vi "read_probes.vi"(8 "error in (no error)":errorcluster, 11 "TempProbeSet in":refnum<class "TempProbeSet.lvclass">) -> (0 "error out":errorcluster, 2 "Array":refnum<class "TempProbe.lvclass">[](array[class]), 3 "TempProbeSet out":refnum<class "TempProbeSet.lvclass">)   [LabVIEW 2010, in "TempProbeSet.lvclass"]
uses:
  TempProbeSet.lvclass
  TempProbe.lvclass
  TempProbeSet.lvclass/TempProbeSet.ctl
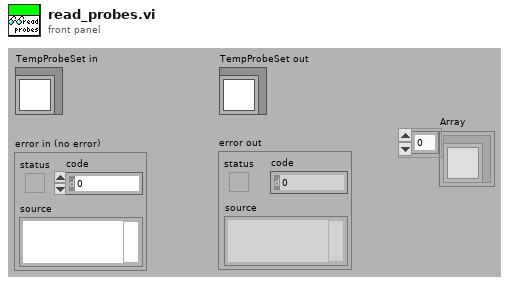
[diagram p1: front panel]
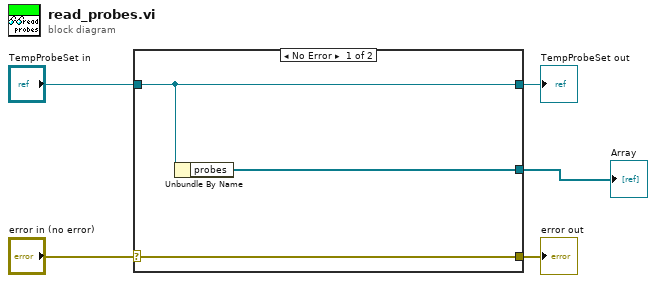
[diagram p0: block diagram]
diagram:
  n1 = case shown="No Error" "error in (no error)" {
    selector: "error in (no error)" -> [w8 w9]
    tunnel: [w8 w9] -> w4
    tunnel: [w7 w10] -> w2
    tunnel: "TempProbeSet in" -> [w7 w10]
    tunnel: [w6 _] -> w1
    frame No Error {
      n2 = Unbundle By Name(w7) -> ("probes"=w6:refnum<class "TempProbe.lvclass">[])
    }
    frame Error {
    }
  }
  "error out" <- w4
  "TempProbeSet out" <- w2
  "Array" <- w1
